vi "MAV_CMD_DO_REPEAT_SERVO.vi"(7 "Cycle Time (s)":sgl, 8 "Cycles":sgl, 9 "PWM (1000 to 2000)":sgl, 10 "Servo Number":sgl, 11 "Target System and Target Component":u8=1) -> (3 "MAVLink Message":u8[](array[numeric]))   [LabVIEW 2014]
panel:
  out "Payload Size":i32
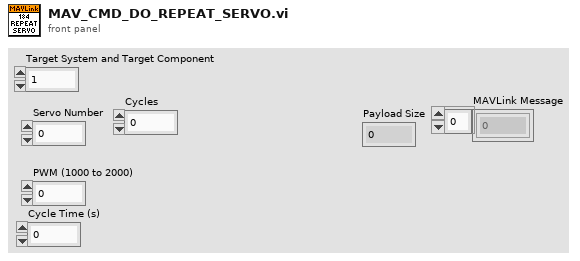
[diagram p1: front panel]
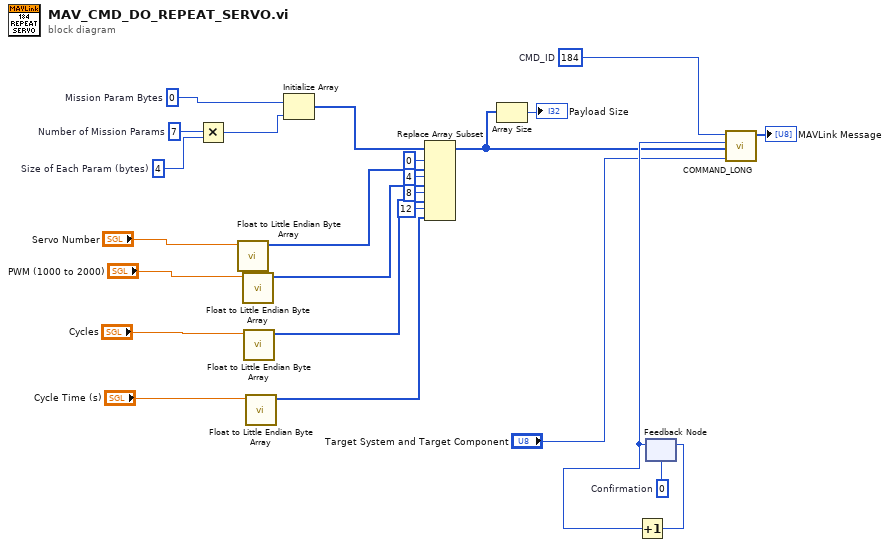
[diagram p0: block diagram]
diagram:
  w18 = u8 0  # Confirmation
  w23 = 4  # Size of Each Param (bytes)
  w24 = 7  # Number of Mission Params
  w25 = u8 0  # Mission Param Bytes
  w14 = u16 184  # CMD_ID
  n1 = Multiply(x=w24, y=w23) -> (x*y=w22:i32)
  n2 = call "Float to Little Endian Byte Array.vi"("Float In"="Servo Number") -> ("LE Byte Array"=w15:u8[])  [unwired: 10 in]
  n3 = call "Float to Little Endian Byte Array.vi"("Float In"="PWM (1000 to 2000)") -> ("LE Byte Array"=w8:u8[])  [unwired: 10 in]
  n4 = call "Float to Little Endian Byte Array.vi"("Float In"="Cycles") -> ("LE Byte Array"=w5:u8[])  [unwired: 10 in]
  n5 = call "Float to Little Endian Byte Array.vi"("Float In"="Cycle Time (s)") -> ("LE Byte Array"=w3:u8[])  [unwired: 10 in]
  n6 = Initialize Array(w25, w22) -> (w21:u8[])
  n7 = Replace Array Subset(array=w21, new element #1=w15, index #1=0 ("index"), new element #2=w8, index #2=4 ("index"), new element #3=w5, index #3=8 ("index"), new element #4=w3, index #4=12 ("index")) -> (w12:u8[])
  n8 = Array Size(array=w12) -> (size(s)=→"Payload Size":i32)
  n9 = feedback #1(w18) -> (w13:u8)
  n10 = Increment(x=w13) -> (x+1=w17:u8)
  n11 = feedback-in #1(w17) -> ()
  n12 = call "COMMAND_LONG.vi"("Target System and Target Component"="Target System and Target Component", "Mission Params"=w12, "Confirmation"=w13, "Command ID"=w14) -> ("MAVLink Message"=→"MAVLink Message":u8[])  [unwired: 7 in]
